vi "DiffertialOdometryAccumalator.vi"(0 "Position":dbl, 1 "Initial Offset":cluster{"X":dbl, "Y":dbl}, 2 "Heading (rad)":dbl, 3 "Reset?":bool) -> (5 "X":dbl, 6 "Y":dbl)   [LabVIEW 2018]
uses:
  <vilib>/Analysis/coordinate.llb/2D Cartesian Coordinate Rotation (Scalar).vi
  <vilib>/Analysis/NI_AALPro.lvlib
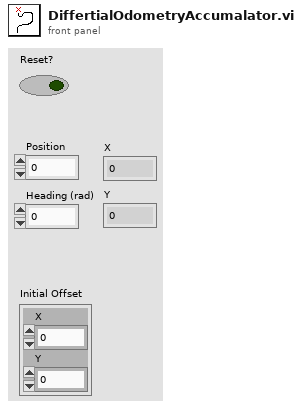
[diagram p1: front panel]
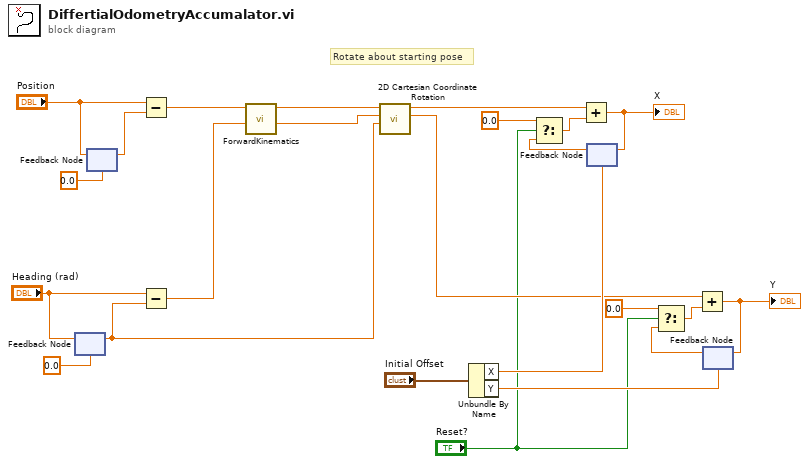
[diagram p0: block diagram]
diagram:
  # "Rotate about starting pose"
  n1 = feedback #1(0.0 ("Heading")) -> (w1:dbl)
  n2 = feedback-in #1("Heading (rad)") -> ()
  n3 = feedback-in #2("Position") -> ()
  n4 = feedback #2(0.0 ("Position")) -> (w22:dbl)
  n5 = Subtract(x="Position", y=w22) -> (x-y=w6:dbl)
  n6 = Subtract(x="Heading (rad)", y=w1) -> (x-y=w3:dbl)
  n7 = call "ForwardKinematics.vi"("dHeading (rad)"=w3, "dX"=w6) -> ("dY"=w4:dbl, "dX"=w5:dbl)  [unwired: 8 in]
  n8 = call-poly <vilib>:"2D Cartesian Coordinate Rotation.vi"("theta"=w1, "y"=w4, "x"=w5) -> ("y out"=w14:dbl, "x out"=w15:dbl)  [unwired: 6 in, 1 out]
  n9 = Unbundle By Name("Initial Offset") -> ("X"=w17:dbl, "Y"=w16:dbl)
  n10 = feedback #3(w17) -> (w12:dbl)
  n11 = Select(t=0.0, s="Reset?", f=w12) -> (s? t:f=w13:dbl)
  n12 = Add(x=w15, y=w13) -> (x+y=w19:dbl)
  "X" <- w19
  n13 = feedback-in #3(w19) -> ()
  n14 = feedback #4(w16) -> (w10:dbl)
  n15 = Select(t=0.0, s="Reset?", f=w10) -> (s? t:f=w9:dbl)
  n16 = Add(x=w14, y=w9) -> (x+y=w20:dbl)
  "Y" <- w20
  n17 = feedback-in #4(w20) -> ()
